vi "Insert into queue.vi"(2 "When did you stick it in?":dbl, 3 "Cell Settings Array":T1(array[cluster])=[{"Measure?"=TRUE, "Area (cm^2)"=0.0, "Cell Label"="", "Cell Description"="", "Time between scans (min)"=0.0, "Cell Position"=0, "Scan settings in queue"=0}, {"Measure?"=TRUE, "Area (cm^2)"=0.0, "Cell Label"="", "Cell Description"="", "Time between scans (min)"=0.0, "Cell Position"=0, "Scan settings in queue"=0}, {"Measure?"=TRUE, "Area (cm^2)"=0.0, "Cell Label"="", "Cell Description"="", "Time between scans (min)"=0.0, "Cell Position"=0, "Scan settings in queue"=0}, {"Measure?"=TRUE, "Area (cm^2)"=0.0, "Cell Label"="", "Cell Description"="", "Time between scans (min)"=0.0, "Cell Position"=0, "Scan settings in queue"=0}, {"Measure?"=TRUE, "Area (cm^2)"=0.0, "Cell Label"="", "Cell Description"="", "Time between scans (min)"=0.0, "Cell Position"=0, "Scan settings in queue"=0}, {"Measure?"=TRUE, "Area (cm^2)"=0.0, "Cell Label"="", "Cell Description"="", "Time between scans (min)"=0.0, "Cell Position"=0, "Scan settings in queue"=0}, {"Measure?"=TRUE, "Area (cm^2)"=0.0, "Cell Label"="", "Cell Description"="", "Time between scans (min)"=0.0, "Cell Position"=0, "Scan settings in queue"=0}, {"Measure?"=TRUE, "Area (cm^2)"=0.0, "Cell Label"="", "Cell Description"="", "Time between scans (min)"=0.0, "Cell Position"=0, "Scan settings in queue"=0}, {"Measure?"=TRUE, "Area (cm^2)"=0.0, "Cell Label"="", "Cell Description"="", "Time between scans (min)"=0.0, "Cell Position"=0, "Scan settings in queue"=0}, {"Measure?"=TRUE, "Area (cm^2)"=0.0, "Cell Label"="", "Cell Description"="", "Time between scans (min)"=0.0, "Cell Position"=0, "Scan settings in queue"=0}, {"Measure?"=TRUE, "Area (cm^2)"=0.0, "Cell Label"="", "Cell Description"="", "Time between scans (min)"=0.0, "Cell Position"=0, "Scan settings in queue"=0}, {"Measure?"=TRUE, "Area (cm^2)"=0.0, "Cell Label"="", "Cell Description"="", "Time between scans (min)"=0.0, "Cell Position"=0, "Scan settings in queue"=0}, {"Measure?"=TRUE, "Area (cm^2)"=0.0, "Cell Label"="", "Cell Description"="", "Time between scans (min)"=0.0, "Cell Position"=0, "Scan settings in queue"=0}, {"Measure?"=TRUE, "Area (cm^2)"=0.0, "Cell Label"="", "Cell Description"="", "Time between scans (min)"=0.0, "Cell Position"=0, "Scan settings in queue"=0}, {"Measure?"=TRUE, "Area (cm^2)"=0.0, "Cell Label"="", "Cell Description"="", "Time between scans (min)"=0.0, "Cell Position"=0, "Scan settings in queue"=0}, {"Measure?"=TRUE, "Area (cm^2)"=0.0, "Cell Label"="", "Cell Description"="", "Time between scans (min)"=0.0, "Cell Position"=0, "Scan settings in queue"=0}] {"Scan settings in queue" items=["Regular", "Inverted"]}, 4 "Queue In":T2(array[cluster])=[{"Measure?"=TRUE, "Area (cm^2)"=0.0, "Cell Label"="", "Cell Description"="", "Cell Position"=0, "Time in rig (h)"=0.0, "Time to next scan (min)"=0.0, "Scan number"=0.0, "When did you stick it in?"=0.0, "Time between scans (min)"=0.0, "Time of the last scan(min)"=0.0, "Scan settings in queue"=0}, {"Measure?"=TRUE, "Area (cm^2)"=0.0, "Cell Label"="", "Cell Description"="", "Cell Position"=0, "Time in rig (h)"=0.0, "Time to next scan (min)"=0.0, "Scan number"=0.0, "When did you stick it in?"=0.0, "Time between scans (min)"=0.0, "Time of the last scan(min)"=0.0, "Scan settings in queue"=0}, {"Measure?"=TRUE, "Area (cm^2)"=0.0, "Cell Label"="", "Cell Description"="", "Cell Position"=0, "Time in rig (h)"=0.0, "Time to next scan (min)"=0.0, "Scan number"=0.0, "When did you stick it in?"=0.0, "Time between scans (min)"=0.0, "Time of the last scan(min)"=0.0, "Scan settings in queue"=0}, {"Measure?"=TRUE, "Area (cm^2)"=0.0, "Cell Label"="", "Cell Description"="", "Cell Position"=0, "Time in rig (h)"=0.0, "Time to next scan (min)"=0.0, "Scan number"=0.0, "When did you stick it in?"=0.0, "Time between scans (min)"=0.0, "Time of the last scan(min)"=0.0, "Scan settings in queue"=0}, {"Measure?"=TRUE, "Area (cm^2)"=0.0, "Cell Label"="", "Cell Description"="", "Cell Position"=0, "Time in rig (h)"=0.0, "Time to next scan (min)"=0.0, "Scan number"=0.0, "When did you stick it in?"=0.0, "Time between scans (min)"=0.0, "Time of the last scan(min)"=0.0, "Scan settings in queue"=0}, {"Measure?"=TRUE, "Area (cm^2)"=0.0, "Cell Label"="", "Cell Description"="", "Cell Position"=0, "Time in rig (h)"=0.0, "Time to next scan (min)"=0.0, "Scan number"=0.0, "When did you stick it in?"=0.0, "Time between scans (min)"=0.0, "Time of the last scan(min)"=0.0, "Scan settings in queue"=0}, {"Measure?"=TRUE, "Area (cm^2)"=0.0, "Cell Label"="", "Cell Description"="", "Cell Position"=0, "Time in rig (h)"=0.0, "Time to next scan (min)"=0.0, "Scan number"=0.0, "When did you stick it in?"=0.0, "Time between scans (min)"=0.0, "Time of the last scan(min)"=0.0, "Scan settings in queue"=0}, {"Measure?"=TRUE, "Area (cm^2)"=0.0, "Cell Label"="", "Cell Description"="", "Cell Position"=0, "Time in rig (h)"=0.0, "Time to next scan (min)"=0.0, "Scan number"=0.0, "When did you stick it in?"=0.0, "Time between scans (min)"=0.0, "Time of the last scan(min)"=0.0, "Scan settings in queue"=0}, {"Measure?"=TRUE, "Area (cm^2)"=0.0, "Cell Label"="", "Cell Description"="", "Cell Position"=0, "Time in rig (h)"=0.0, "Time to next scan (min)"=0.0, "Scan number"=0.0, "When did you stick it in?"=0.0, "Time between scans (min)"=0.0, "Time of the last scan(min)"=0.0, "Scan settings in queue"=0}, {"Measure?"=TRUE, "Area (cm^2)"=0.0, "Cell Label"="", "Cell Description"="", "Cell Position"=0, "Time in rig (h)"=0.0, "Time to next scan (min)"=0.0, "Scan number"=0.0, "When did you stick it in?"=0.0, "Time between scans (min)"=0.0, "Time of the last scan(min)"=0.0, "Scan settings in queue"=0}, {"Measure?"=TRUE, "Area (cm^2)"=0.0, "Cell Label"="", "Cell Description"="", "Cell Position"=0, "Time in rig (h)"=0.0, "Time to next scan (min)"=0.0, "Scan number"=0.0, "When did you stick it in?"=0.0, "Time between scans (min)"=0.0, "Time of the last scan(min)"=0.0, "Scan settings in queue"=0}, {"Measure?"=TRUE, "Area (cm^2)"=0.0, "Cell Label"="", "Cell Description"="", "Cell Position"=0, "Time in rig (h)"=0.0, "Time to next scan (min)"=0.0, "Scan number"=0.0, "When did you stick it in?"=0.0, "Time between scans (min)"=0.0, "Time of the last scan(min)"=0.0, "Scan settings in queue"=0}, {"Measure?"=TRUE, "Area (cm^2)"=0.0, "Cell Label"="", "Cell Description"="", "Cell Position"=0, "Time in rig (h)"=0.0, "Time to next scan (min)"=0.0, "Scan number"=0.0, "When did you stick it in?"=0.0, "Time between scans (min)"=0.0, "Time of the last scan(min)"=0.0, "Scan settings in queue"=0}, {"Measure?"=TRUE, "Area (cm^2)"=0.0, "Cell Label"="", "Cell Description"="", "Cell Position"=0, "Time in rig (h)"=0.0, "Time to next scan (min)"=0.0, "Scan number"=0.0, "When did you stick it in?"=0.0, "Time between scans (min)"=0.0, "Time of the last scan(min)"=0.0, "Scan settings in queue"=0}, {"Measure?"=TRUE, "Area (cm^2)"=0.0, "Cell Label"="", "Cell Description"="", "Cell Position"=0, "Time in rig (h)"=0.0, "Time to next scan (min)"=0.0, "Scan number"=0.0, "When did you stick it in?"=0.0, "Time between scans (min)"=0.0, "Time of the last scan(min)"=0.0, "Scan settings in queue"=0}, {"Measure?"=TRUE, "Area (cm^2)"=0.0, "Cell Label"="", "Cell Description"="", "Cell Position"=0, "Time in rig (h)"=0.0, "Time to next scan (min)"=0.0, "Scan number"=0.0, "When did you stick it in?"=0.0, "Time between scans (min)"=0.0, "Time of the last scan(min)"=0.0, "Scan settings in queue"=0}] {"Scan settings in queue" items=["Regular", "Inverted"]; "Time of the last scan(min)" format="%<%H:%M:%S>t"; "When did you stick it in?" format="%<%H:%M:%S>t"; "Time to next scan (min)" format="%<%H:%M:%S>t"; "Time in rig (h)" format="%<%H:%M:%S>t"}) -> (0 "Queue":T2(array[cluster])=[{"Measure?"=TRUE, "Area (cm^2)"=0.0, "Cell Label"="", "Cell Description"="", "Cell Position"=0, "Time in rig (h)"=0.0, "Time to next scan (min)"=0.0, "Scan number"=0.0, "When did you stick it in?"=0.0, "Time between scans (min)"=0.0, "Time of the last scan(min)"=0.0, "Scan settings in queue"=0}, {"Measure?"=TRUE, "Area (cm^2)"=0.0, "Cell Label"="", "Cell Description"="", "Cell Position"=0, "Time in rig (h)"=0.0, "Time to next scan (min)"=0.0, "Scan number"=0.0, "When did you stick it in?"=0.0, "Time between scans (min)"=0.0, "Time of the last scan(min)"=0.0, "Scan settings in queue"=0}, {"Measure?"=TRUE, "Area (cm^2)"=0.0, "Cell Label"="", "Cell Description"="", "Cell Position"=0, "Time in rig (h)"=0.0, "Time to next scan (min)"=0.0, "Scan number"=0.0, "When did you stick it in?"=0.0, "Time between scans (min)"=0.0, "Time of the last scan(min)"=0.0, "Scan settings in queue"=0}, {"Measure?"=TRUE, "Area (cm^2)"=0.0, "Cell Label"="", "Cell Description"="", "Cell Position"=0, "Time in rig (h)"=0.0, "Time to next scan (min)"=0.0, "Scan number"=0.0, "When did you stick it in?"=0.0, "Time between scans (min)"=0.0, "Time of the last scan(min)"=0.0, "Scan settings in queue"=0}, {"Measure?"=TRUE, "Area (cm^2)"=0.0, "Cell Label"="", "Cell Description"="", "Cell Position"=0, "Time in rig (h)"=0.0, "Time to next scan (min)"=0.0, "Scan number"=0.0, "When did you stick it in?"=0.0, "Time between scans (min)"=0.0, "Time of the last scan(min)"=0.0, "Scan settings in queue"=0}, {"Measure?"=TRUE, "Area (cm^2)"=0.0, "Cell Label"="", "Cell Description"="", "Cell Position"=0, "Time in rig (h)"=0.0, "Time to next scan (min)"=0.0, "Scan number"=0.0, "When did you stick it in?"=0.0, "Time between scans (min)"=0.0, "Time of the last scan(min)"=0.0, "Scan settings in queue"=0}, {"Measure?"=TRUE, "Area (cm^2)"=0.0, "Cell Label"="", "Cell Description"="", "Cell Position"=0, "Time in rig (h)"=0.0, "Time to next scan (min)"=0.0, "Scan number"=0.0, "When did you stick it in?"=0.0, "Time between scans (min)"=0.0, "Time of the last scan(min)"=0.0, "Scan settings in queue"=0}, {"Measure?"=TRUE, "Area (cm^2)"=0.0, "Cell Label"="", "Cell Description"="", "Cell Position"=0, "Time in rig (h)"=0.0, "Time to next scan (min)"=0.0, "Scan number"=0.0, "When did you stick it in?"=0.0, "Time between scans (min)"=0.0, "Time of the last scan(min)"=0.0, "Scan settings in queue"=0}, {"Measure?"=TRUE, "Area (cm^2)"=0.0, "Cell Label"="", "Cell Description"="", "Cell Position"=0, "Time in rig (h)"=0.0, "Time to next scan (min)"=0.0, "Scan number"=0.0, "When did you stick it in?"=0.0, "Time between scans (min)"=0.0, "Time of the last scan(min)"=0.0, "Scan settings in queue"=0}, {"Measure?"=TRUE, "Area (cm^2)"=0.0, "Cell Label"="", "Cell Description"="", "Cell Position"=0, "Time in rig (h)"=0.0, "Time to next scan (min)"=0.0, "Scan number"=0.0, "When did you stick it in?"=0.0, "Time between scans (min)"=0.0, "Time of the last scan(min)"=0.0, "Scan settings in queue"=0}, {"Measure?"=TRUE, "Area (cm^2)"=0.0, "Cell Label"="", "Cell Description"="", "Cell Position"=0, "Time in rig (h)"=0.0, "Time to next scan (min)"=0.0, "Scan number"=0.0, "When did you stick it in?"=0.0, "Time between scans (min)"=0.0, "Time of the last scan(min)"=0.0, "Scan settings in queue"=0}, {"Measure?"=TRUE, "Area (cm^2)"=0.0, "Cell Label"="", "Cell Description"="", "Cell Position"=0, "Time in rig (h)"=0.0, "Time to next scan (min)"=0.0, "Scan number"=0.0, "When did you stick it in?"=0.0, "Time between scans (min)"=0.0, "Time of the last scan(min)"=0.0, "Scan settings in queue"=0}, {"Measure?"=TRUE, "Area (cm^2)"=0.0, "Cell Label"="", "Cell Description"="", "Cell Position"=0, "Time in rig (h)"=0.0, "Time to next scan (min)"=0.0, "Scan number"=0.0, "When did you stick it in?"=0.0, "Time between scans (min)"=0.0, "Time of the last scan(min)"=0.0, "Scan settings in queue"=0}, {"Measure?"=TRUE, "Area (cm^2)"=0.0, "Cell Label"="", "Cell Description"="", "Cell Position"=0, "Time in rig (h)"=0.0, "Time to next scan (min)"=0.0, "Scan number"=0.0, "When did you stick it in?"=0.0, "Time between scans (min)"=0.0, "Time of the last scan(min)"=0.0, "Scan settings in queue"=0}, {"Measure?"=TRUE, "Area (cm^2)"=0.0, "Cell Label"="", "Cell Description"="", "Cell Position"=0, "Time in rig (h)"=0.0, "Time to next scan (min)"=0.0, "Scan number"=0.0, "When did you stick it in?"=0.0, "Time between scans (min)"=0.0, "Time of the last scan(min)"=0.0, "Scan settings in queue"=0}, {"Measure?"=TRUE, "Area (cm^2)"=0.0, "Cell Label"="", "Cell Description"="", "Cell Position"=0, "Time in rig (h)"=0.0, "Time to next scan (min)"=0.0, "Scan number"=0.0, "When did you stick it in?"=0.0, "Time between scans (min)"=0.0, "Time of the last scan(min)"=0.0, "Scan settings in queue"=0}] {"Scan settings in queue" items=["Regular", "Inverted"]; "Time of the last scan(min)" format="%<%H:%M:%S>t"; "When did you stick it in?" format="%<%H:%M:%S>t"; "Time to next scan (min)" format="%<%H:%M:%S>t"; "Time in rig (h)" format="%<%H:%M:%S>t"}, 1 "Cell Settings Array 2":T1(array[cluster])=[{"Measure?"=TRUE, "Area (cm^2)"=0.0, "Cell Label"="", "Cell Description"="", "Time between scans (min)"=0.0, "Cell Position"=0, "Scan settings in queue"=0}, {"Measure?"=TRUE, "Area (cm^2)"=0.0, "Cell Label"="", "Cell Description"="", "Time between scans (min)"=0.0, "Cell Position"=0, "Scan settings in queue"=0}, {"Measure?"=TRUE, "Area (cm^2)"=0.0, "Cell Label"="", "Cell Description"="", "Time between scans (min)"=0.0, "Cell Position"=0, "Scan settings in queue"=0}, {"Measure?"=TRUE, "Area (cm^2)"=0.0, "Cell Label"="", "Cell Description"="", "Time between scans (min)"=0.0, "Cell Position"=0, "Scan settings in queue"=0}, {"Measure?"=TRUE, "Area (cm^2)"=0.0, "Cell Label"="", "Cell Description"="", "Time between scans (min)"=0.0, "Cell Position"=0, "Scan settings in queue"=0}, {"Measure?"=TRUE, "Area (cm^2)"=0.0, "Cell Label"="", "Cell Description"="", "Time between scans (min)"=0.0, "Cell Position"=0, "Scan settings in queue"=0}, {"Measure?"=TRUE, "Area (cm^2)"=0.0, "Cell Label"="", "Cell Description"="", "Time between scans (min)"=0.0, "Cell Position"=0, "Scan settings in queue"=0}, {"Measure?"=TRUE, "Area (cm^2)"=0.0, "Cell Label"="", "Cell Description"="", "Time between scans (min)"=0.0, "Cell Position"=0, "Scan settings in queue"=0}, {"Measure?"=TRUE, "Area (cm^2)"=0.0, "Cell Label"="", "Cell Description"="", "Time between scans (min)"=0.0, "Cell Position"=0, "Scan settings in queue"=0}, {"Measure?"=TRUE, "Area (cm^2)"=0.0, "Cell Label"="", "Cell Description"="", "Time between scans (min)"=0.0, "Cell Position"=0, "Scan settings in queue"=0}, {"Measure?"=TRUE, "Area (cm^2)"=0.0, "Cell Label"="", "Cell Description"="", "Time between scans (min)"=0.0, "Cell Position"=0, "Scan settings in queue"=0}, {"Measure?"=TRUE, "Area (cm^2)"=0.0, "Cell Label"="", "Cell Description"="", "Time between scans (min)"=0.0, "Cell Position"=0, "Scan settings in queue"=0}, {"Measure?"=TRUE, "Area (cm^2)"=0.0, "Cell Label"="", "Cell Description"="", "Time between scans (min)"=0.0, "Cell Position"=0, "Scan settings in queue"=0}, {"Measure?"=TRUE, "Area (cm^2)"=0.0, "Cell Label"="", "Cell Description"="", "Time between scans (min)"=0.0, "Cell Position"=0, "Scan settings in queue"=0}, {"Measure?"=TRUE, "Area (cm^2)"=0.0, "Cell Label"="", "Cell Description"="", "Time between scans (min)"=0.0, "Cell Position"=0, "Scan settings in queue"=0}, {"Measure?"=TRUE, "Area (cm^2)"=0.0, "Cell Label"="", "Cell Description"="", "Time between scans (min)"=0.0, "Cell Position"=0, "Scan settings in queue"=0}] {"Scan settings in queue" items=["Regular", "Inverted"]})   [LabVIEW 2011]
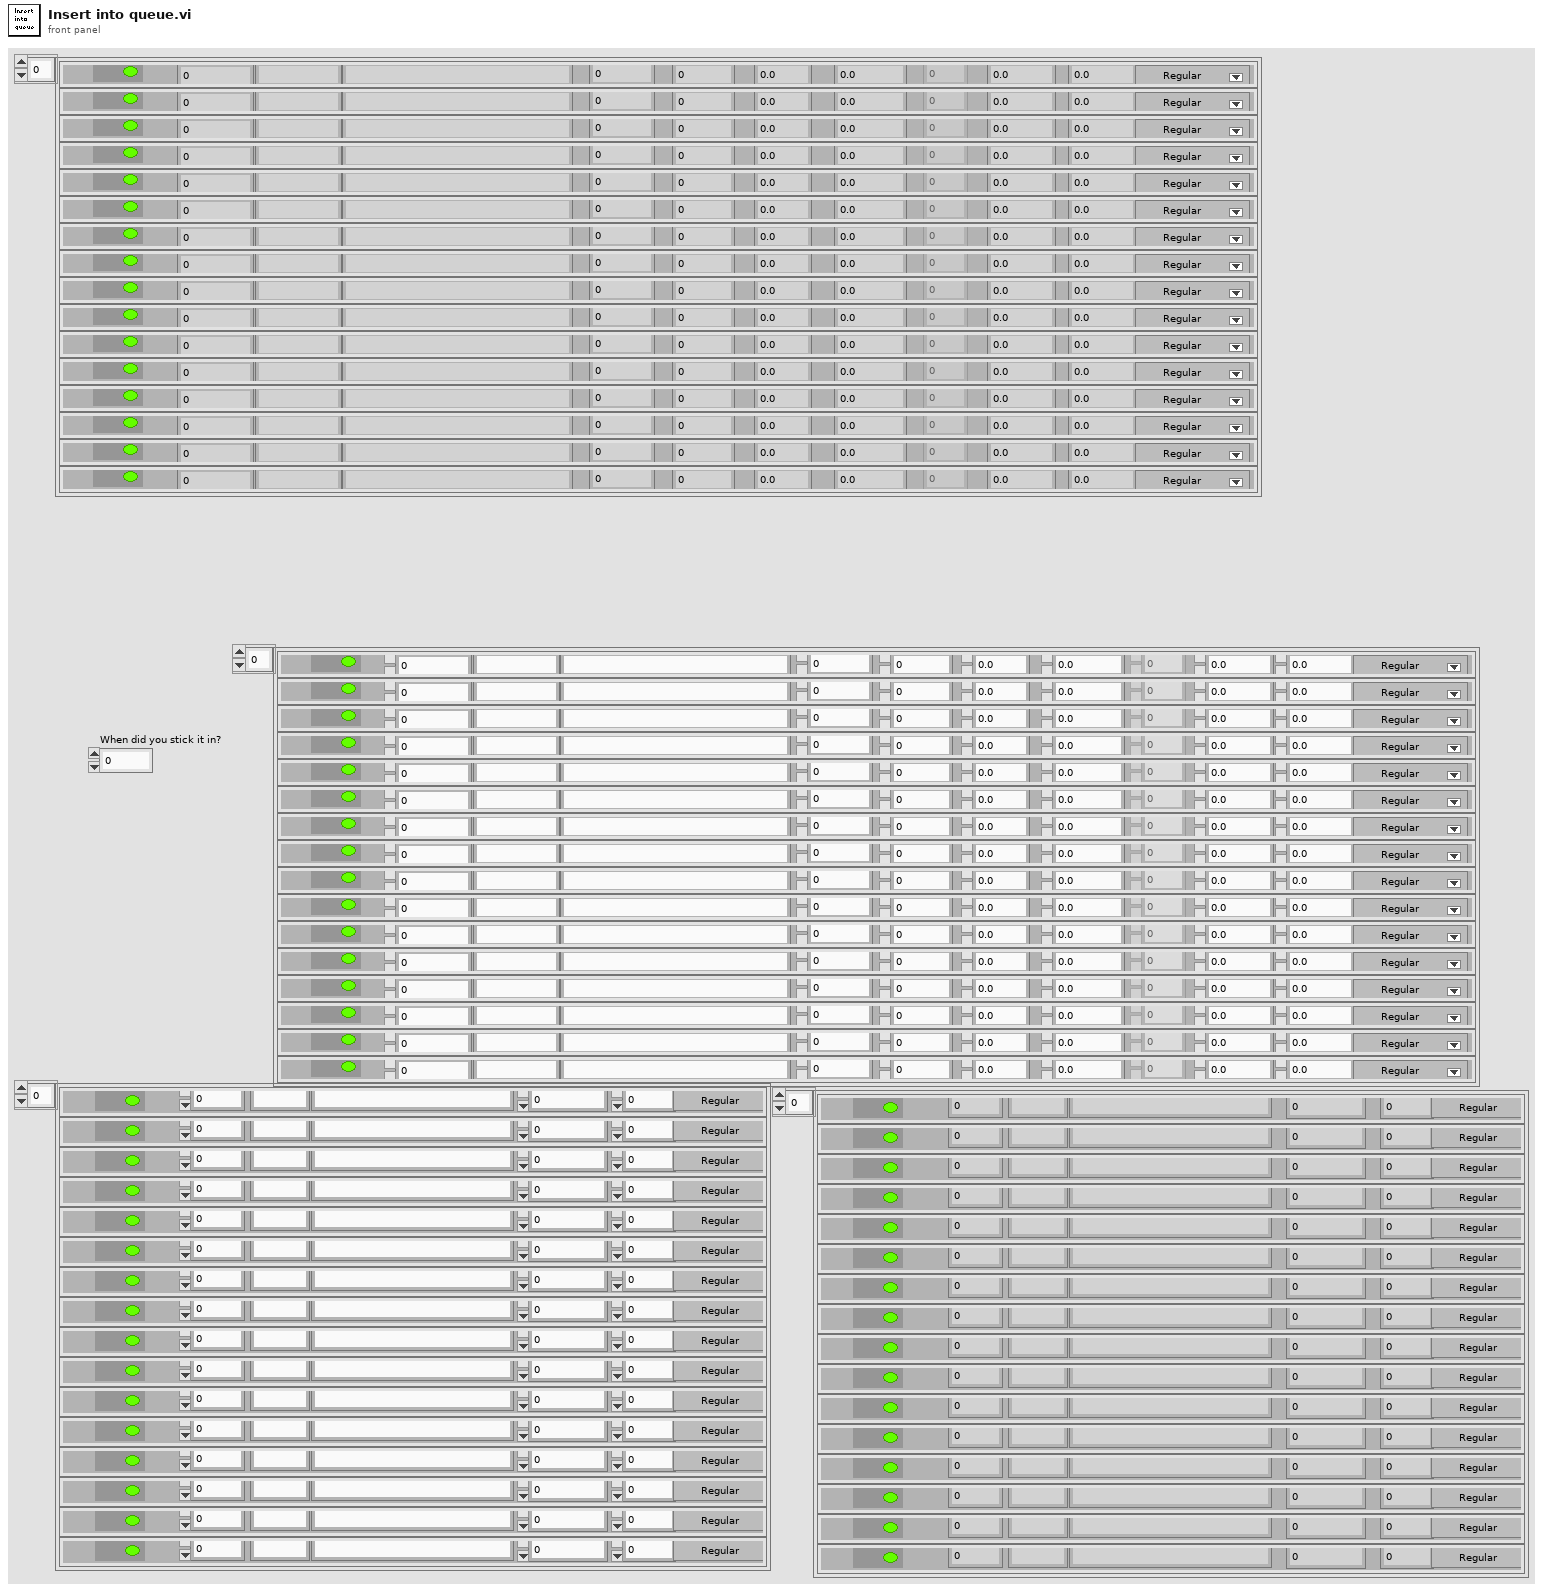
[diagram p1: front panel]
types:
  T1 = cluster{"Measure?":bool, "Area (cm^2)":dbl, "Cell Label":string, "Cell Description":string, "Time between scans (min)":dbl, "Cell Position":i32, "Scan settings in queue":u16}[]
  T2 = cluster{"Measure?":bool, "Area (cm^2)":dbl, "Cell Label":string, "Cell Description":string, "Cell Position":i32, "Time in rig (h)":dbl, "Time to next scan (min)":dbl, "Scan number":dbl, "When did you stick it in?":dbl, "Time between scans (min)":dbl, "Time of the last scan(min)":dbl, "Scan settings in queue":u16}[]
  T3 = cluster{"Measure?":bool, "Area (cm^2)":dbl, "Cell Label":string, "Cell Description":string, "Cell Position":i32, "Time in rig (h)":dbl, "Time to next scan (min)":dbl, "Scan number":dbl, "When did you stick it in?":dbl, "Time between scans (min)":dbl, "Time of the last scan(min)":dbl, "Scan settings in queue":u16}
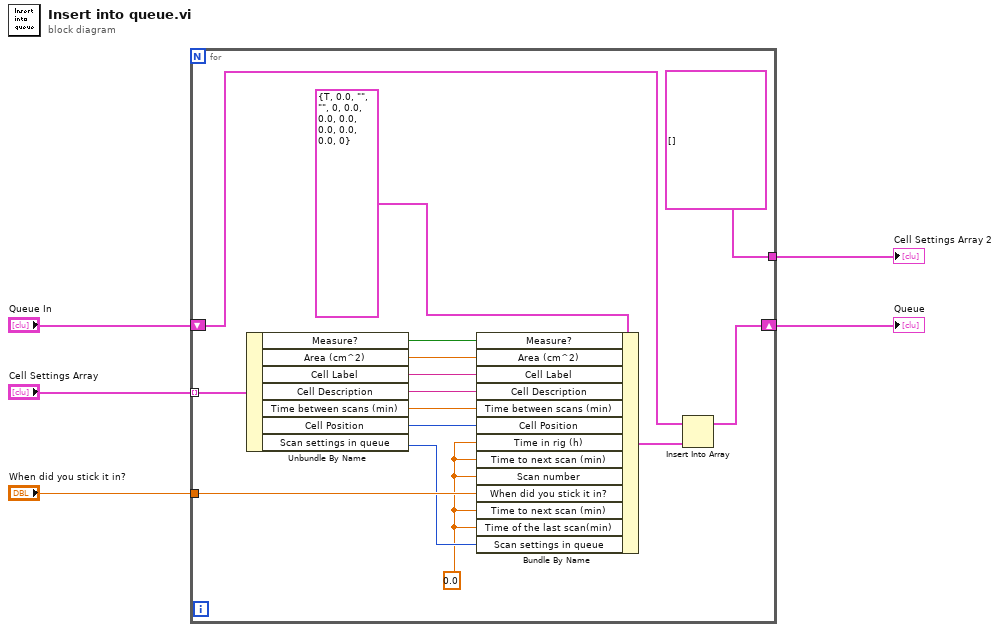
[diagram p0: block diagram]
diagram:
  n1 = for {
    tunnel: "Cell Settings Array" -> [w15] mode=indexing
    tunnel: "When did you stick it in?" -> [w16]
    shift-right: [w10] -> w3
    shift-left: "Queue In" -> [w12]
    tunnel: [T1 [] ("Cell Settings Array 2")] -> w1
    w6 = 0.0 ("Time of the last scan (min)")
    n2 = Unbundle By Name(w15) -> ("Measure?"=w14:bool, "Area (cm^2)"=w13:dbl, "Cell Label"=w20:string, "Cell Description"=w19:string, "Time between scans (min)"=w18:dbl, "Cell Position"=w17:i32, "Scan settings in queue"=w7:u16)
    n3 = Bundle By Name(cluster=T3 {"Measure?"=TRUE, "Area (cm^2)"=0.0, "Cell Label"="", "Cell Description"="", "Cell Position"=0, "Time in rig (h)"=0.0, "Time to next scan (min)"=0.0, "Scan number"=0.0, "When did you stick it in?"=0.0, "Time between scans (min)"=0.0, "Time of the last scan(min)"=0.0, "Scan settings in queue"=0} ("Cluster"), "Measure?"=w14, "Area (cm^2)"=w13, "Cell Label"=w20, "Cell Description"=w19, "Time between scans (min)"=w18, "Cell Position"=w17, "Time in rig (h)"=w6, "Time to next scan (min)"=w6, "Scan number"=w6, "When did you stick it in?"=w16, "Time to next scan (min)"=w6, "Time of the last scan(min)"=w6, "Scan settings in queue"=w7) -> (w11:T3)
    n4 = Insert Into Array(array=w12, new element=w11) -> (w10:T2)  [unwired: 1 in]
  }
  "Queue" <- w3
  "Cell Settings Array 2" <- w1
